vi "DAQ_pressure_flow_subVI.vi"(0 "vac press":dbl[](array[numeric])) -> (2 "Cluster 2":cluster{"f":dbl, "f":dbl}, 3 "pressure":dbl, 6 "vapor flow":dbl, 10 "press/RH/gas/vapor":T1, 15 "gas flow":dbl)   [LabVIEW 2014]
panel:
  out "RH":string
  out "save pressure":string
  out "save gas flow":string
  out "save vapor flow":string
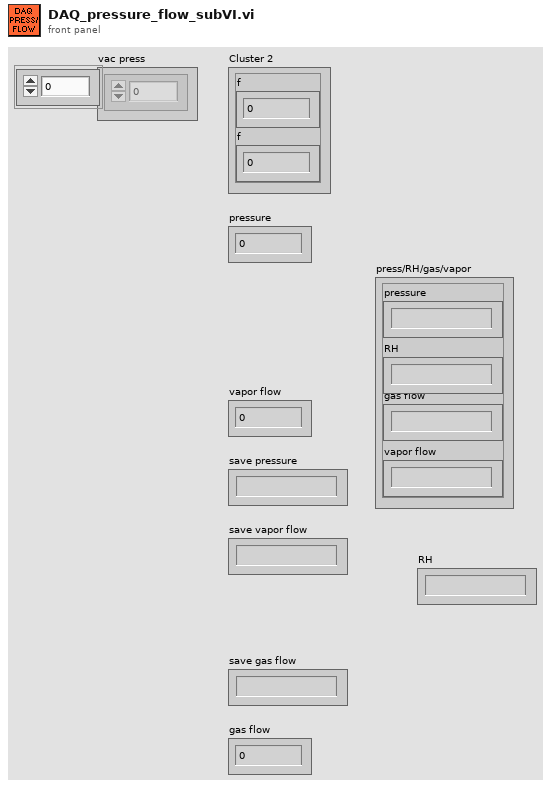
[diagram p1: front panel]
types:
  T1 = cluster{"pressure":string, "RH":string, "gas flow":string, "vapor flow":string}
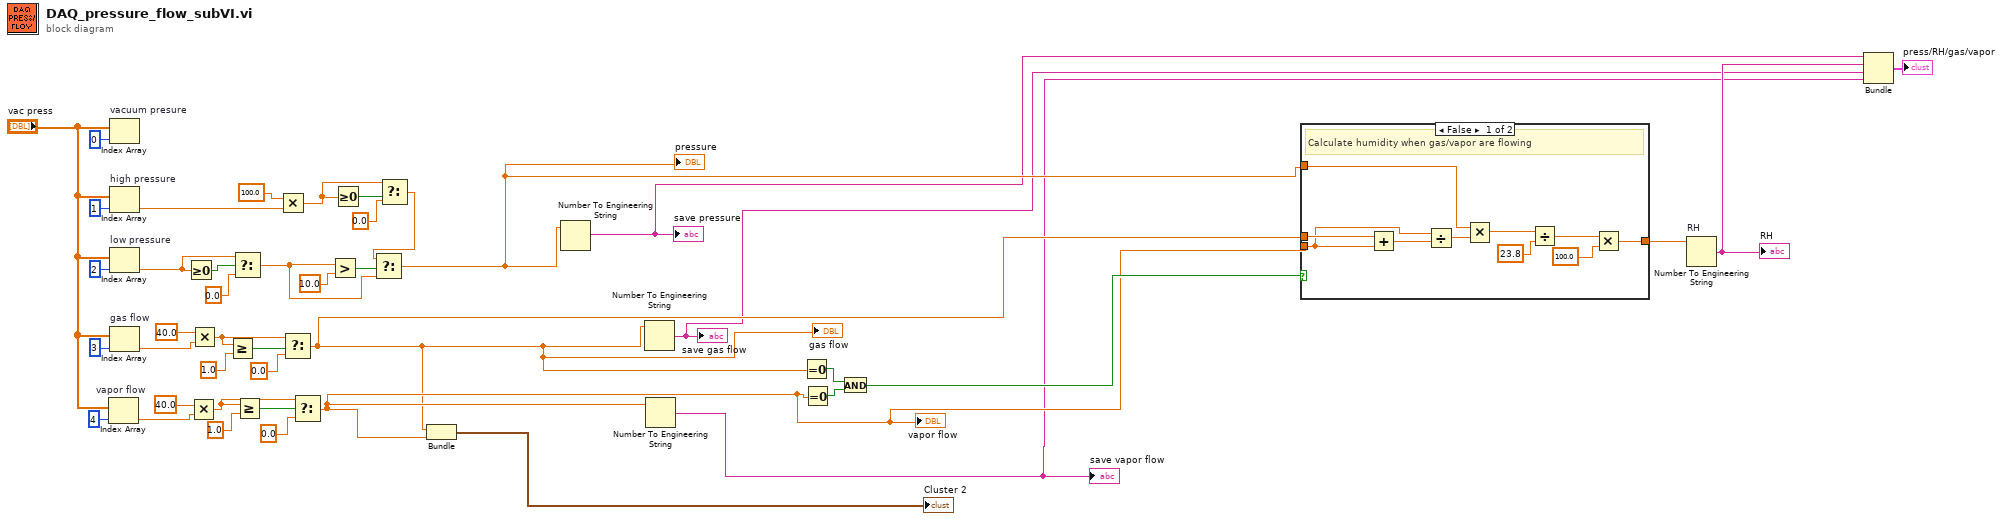
[diagram p0: block diagram]
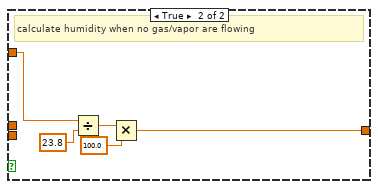
[diagram p2: hidden frame]
diagram:
  n1 = Index Array "vapor flow"(array="vac press", index=4) -> (element=w22:dbl)
  n2 = Index Array "vacuum presure"(array="vac press", index=0) -> ()  [unwired: 1 out]
  n3 = Index Array "high pressure"(array="vac press", index=1) -> (element=w15:dbl)
  n4 = Index Array "low pressure"(array="vac press", index=2) -> (element=w39:dbl)
  n5 = Index Array "gas flow"(array="vac press", index=3) -> (element=w20:dbl)
  n6 = Greater Or Equal To 0?(x=w39) -> (x >= 0?=w38:bool)
  n7 = Multiply(x=40.0, y=w22) -> (x*y=w29:dbl)
  n8 = Multiply(x=40.0, y=w20) -> (x*y=w32:dbl)
  n9 = Greater Or Equal?(x=w32, y=1.0) -> (x >= y?=w33:bool)
  n10 = Select(t=w39, s=w38, f=0.0) -> (s? t:f=w40:dbl)
  n11 = Greater Or Equal?(x=w29, y=1.0) -> (x >= y?=w30:bool)
  n12 = Multiply(x=100.0, y=w15) -> (x*y=w27:dbl)
  n13 = Select(t=w32, s=w33, f=0.0) -> (s? t:f=w6:dbl)
  "gas flow" <- w6
  n14 = Select(t=w29, s=w30, f=0.0) -> (s? t:f=w7:dbl)
  "vapor flow" <- w7
  n15 = Greater?(x=w40, y=10.0) -> (0:w35:bool)
  n16 = Greater Or Equal To 0?(x=w27) -> (x >= 0?=w25:bool)
  n17 = Select(t=w27, s=w25, f=0.0) -> (s? t:f=w36:dbl)
  n18 = Select(t=w36, s=w35, f=w40) -> (s? t:f=w9:dbl)
  "pressure" <- w9
  n19 = Bundle("f"=w6, "f"=w7) -> (→"Cluster 2":cluster{"f":dbl, "f":dbl})  [unwired: 1 in]
  n20 = Number To Engineering String(4:w9) -> (0:w5:string)  [unwired: 3 in]
  "save pressure" <- w5
  n21 = Number To Engineering String(4:w6) -> (0:w3:string)  [unwired: 3 in]
  "save gas flow" <- w3
  n22 = Number To Engineering String(4:w7) -> (0:w2:string)  [unwired: 3 in]
  "save vapor flow" <- w2
  n23 = Equal To 0?(x=w6) -> (x = 0?=w43:bool)
  n24 = Equal To 0?(x=w7) -> (x = 0?=w42:bool)
  n25 = And(x=w43, y=w42) -> (x .and. y?=w8:bool)
  n26 = case shown="False" w8 {
    tunnel: w9 -> [w45 w55]
    tunnel: [w44 w54] -> w10
    tunnel: w6 -> [w53 _]
    tunnel: w7 -> [w51 _]
    frame False {
      # "Calculate humidity when gas/vapor are flowing"
      n27 = Add(x=w53, y=w51) -> (x+y=w52:dbl)
      n28 = Divide(x=w51, y=w52) -> (x/y=w46:dbl)
      n29 = Multiply(x=w45, y=w46) -> (x*y=w47:dbl)
      n30 = Divide(x=w47, y=23.8) -> (x/y=w49:dbl)
      n31 = Multiply(x=w49, y=100.0) -> (x*y=w44:dbl)
    }
    frame True {
      # "calculate humidity when no gas/vapor are flowing"
      n32 = Divide(x=w55, y=23.8) -> (x/y=w57:dbl)
      n33 = Multiply(x=w57, y=100.0) -> (x*y=w54:dbl)
    }
  }
  n34 = Number To Engineering String "RH"(4:w10) -> (0:w4:string)  [unwired: 3 in]
  "RH" <- w4
  n35 = Bundle(w5, w4, w3, w2) -> (→"press/RH/gas/vapor":cluster{string, string, string, string})  [unwired: 1 in]
